vi "readCurrent.vi"(6 "error in (no error)":errorcluster, 9 "VISA resource name":refnum<visa-resource-name>) -> (0 "error out":errorcluster, 1 "Corriente":dbl(knob) scale=0.0..10.0, 2 "Voltaje":dbl(knob) scale=0.0..10.0, 3 "VISA Refnum out":refnum<visa-resource-name>, 4 "read buffer":string)   [LabVIEW 2026]
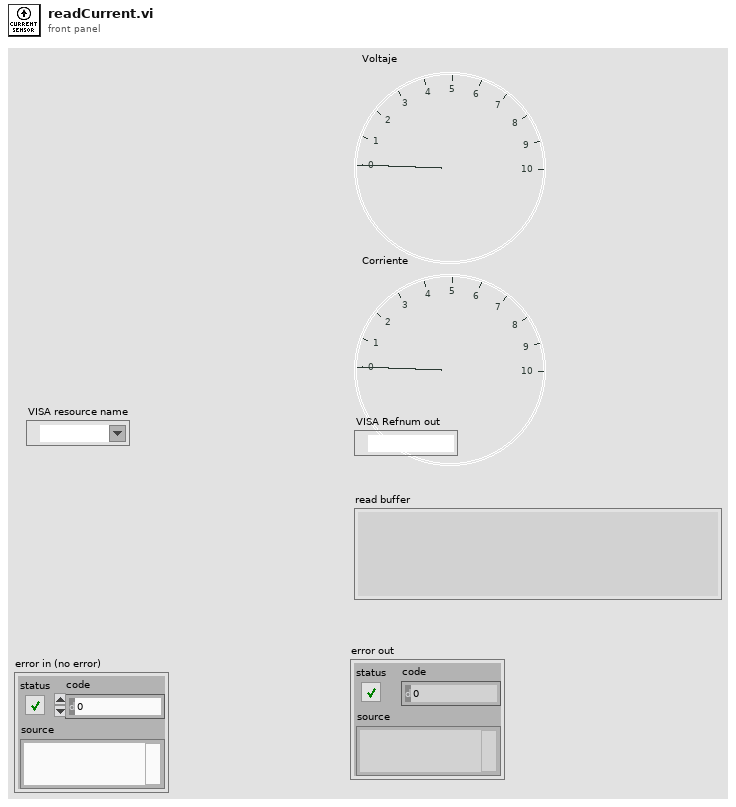
[diagram p1: front panel]
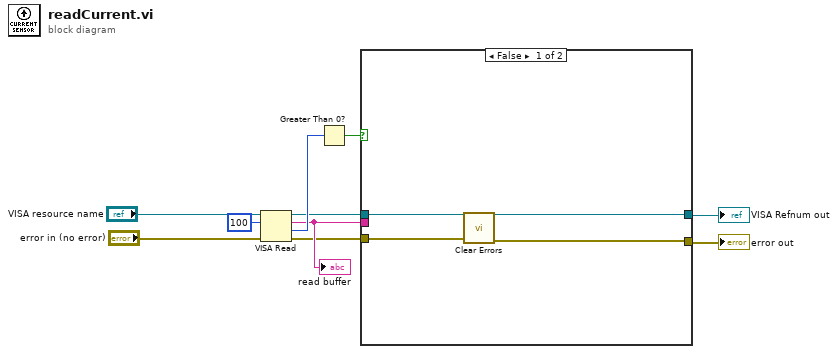
[diagram p0: block diagram]
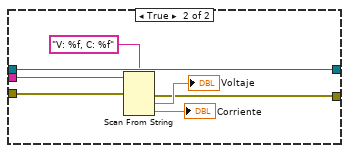
[diagram p2: hidden frame]
diagram:
  n1 = VISA Read(VISA resource name="VISA resource name", byte count=u32 100, error in (no error)="error in (no error)") -> (VISA resource name out=w4:refnum<visa-resource-name>, read buffer=w6:string, return count=w7:u32, error out=w3:errorcluster)
  "read buffer" <- w6
  n2 = Greater Than 0?(x=w7) -> (x > 0?=w8:bool)
  n3 = case shown="False" w8 {
    tunnel: w3 -> [w13 w16]
    tunnel: w4 -> [w11 w20]
    tunnel: [w11 w20] -> w9
    tunnel: [w12 w15] -> w5
    tunnel: w6 -> [_ w14]
    frame False {
      n4 = call <vilib>:"Clear Errors.vi"("error in (no error)"=w13) -> ("error out"=w12:errorcluster)  [unwired: 5 in, 1 out]
    }
    frame True {
      n5 = Scan From String(format string="V: %f, C: %f", input string=w14, error in=w16) -> (error out=w15:errorcluster, output 1=→"Voltaje":dbl, output 2=→"Corriente":dbl)  [unwired: 3 in, 2 out]
    }
  }
  "VISA Refnum out" <- w9
  "error out" <- w5
